vi "BRig_Host__Loop_Consumer_RunState__typeTrial__subtypeSelResult_parse__v2.vi"(0 "input_strCmd":string) -> (3 "output_selResult":bool, 4 "output_nTrial":u16, 6 "output_sSelection":u16, 8 "output_tSelection":u16, 10 "output_iReward_or_iError":u16, 13 "output_trig_l2":u16, 14 "output_trig_l1":u16, 15 "output_LorR":u16)   [LabVIEW 2014]
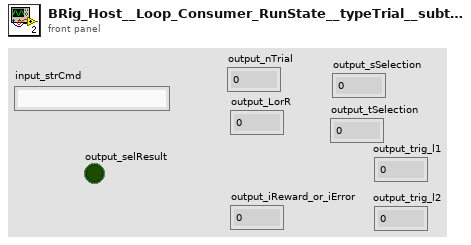
[diagram p1: front panel]
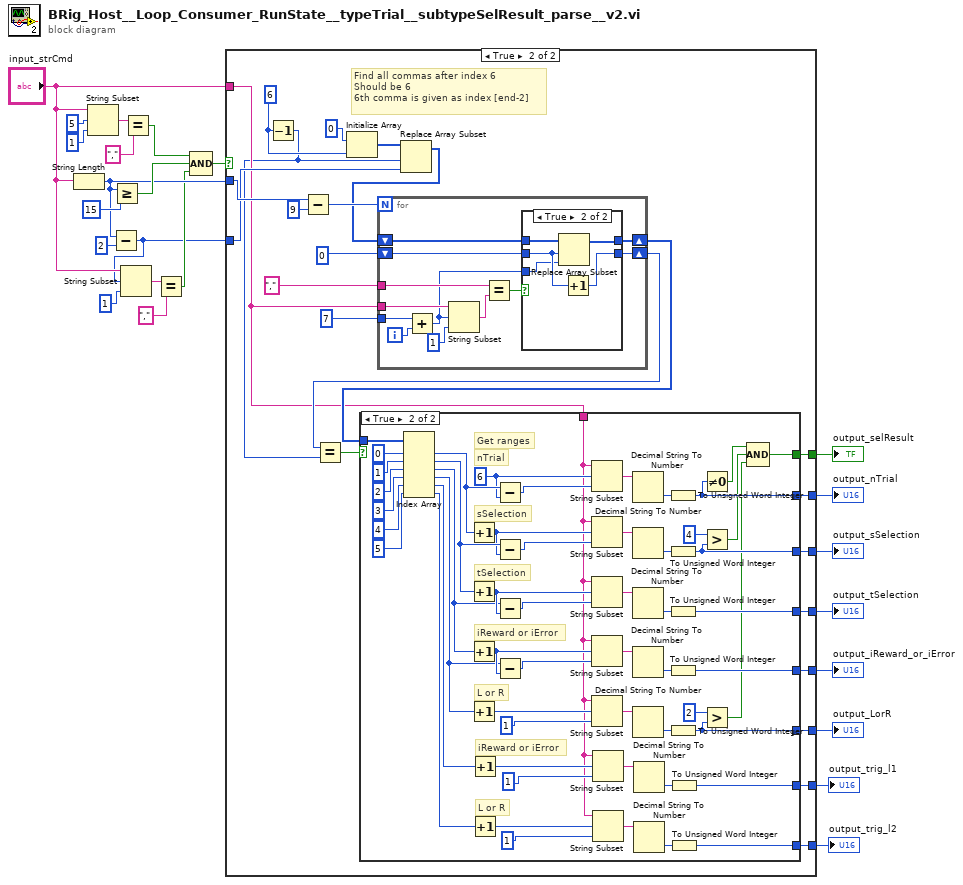
[diagram p0: block diagram]
diagram:
  n1 = String Length(string="input_strCmd") -> (length=w12:i32)
  n2 = String Subset(string="input_strCmd", offset (0)=5, length (rest)=1 ("offset (0)")) -> (substring=w22:string)
  n3 = Subtract(x=w12, y=2) -> (x-y=w9:i32)
  n4 = Greater Or Equal?(x=w12, y=15) -> (x >= y?=w19:bool)
  n5 = String Subset(string="input_strCmd", offset (0)=w9, length (rest)=1 ("offset (0)")) -> (substring=w14:string)
  n6 = Equal?(x=w22, y=",") -> (x = y?=w18:bool)
  n7 = Equal?(x=w14, y=",") -> (x = y?=w10:bool)
  n8 = Compound Arithmetic op=AND(w18, w19, w10) -> (w17:bool)
  n9 = case shown="True" w17 {
    tunnel: "input_strCmd" -> [_ w36]
    tunnel: w12 -> [_ w46]
    tunnel: w9 -> [_ w38]
    tunnel: [_ w34] -> w8
    tunnel: [_ w33] -> w7
    tunnel: [_ w32] -> w6
    tunnel: [_ w31] -> w5
    tunnel: [_ w30] -> w4
    tunnel: [_ w29] -> w3
    tunnel: [_ w26] -> w2
    tunnel: [_ w25] -> w1
    frame False {
    }
    frame True {
      w28 = 6 ("dimension size")
      # "Find all commas after index 6\nShould be 6\n6th comma is given as index [end-2]"
      n10 = Decrement(x=w28) -> (x-1=w27:i32)
      n11 = Subtract(x=w46, y=9) -> (x-y=w45:i32)
      n12 = Initialize Array(0 ("element"), w28) -> (w40:i32[])
      n13 = Replace Array Subset(array=w40, new element=w38, index=w27) -> (w39:i32[])
      n14 = for {
        N: w45 -> [_]
        tunnel: w36 -> [w114]
        tunnel: "," ("y") -> [w112]
        tunnel: 7 ("element") -> [w110]
        shift-right: [w104] -> w41
        shift-left: 0 ("element") -> [w106]
        shift-right: [w105] -> w37
        shift-left: w39 -> [w107]
        i -> [w111]
        n15 = Add(x=w110, y=w111) -> (x+y=w108:i32)
        n16 = String Subset(string=w114, offset (0)=w108, length (rest)=1 ("offset (0)")) -> (substring=w113:string)
        n17 = Equal?(x=w112, y=w113) -> (x = y?=w109:bool)
        n18 = case shown="True" w109 {
          tunnel: w108 -> [_ w119]
          tunnel: w107 -> [w117 w122]
          tunnel: w106 -> [w116 w120]
          tunnel: [w117 w121] -> w105
          tunnel: [w116 w118] -> w104
          frame False {
          }
          frame True {
            n19 = Replace Array Subset(array=w122, new element=w119, index=w120) -> (w121:i32[])
            n20 = Increment(x=w120) -> (x+1=w118:i32)
          }
        }
      }
      n21 = Equal?(x=w41, y=w27) -> (x = y?=w35:bool)
      n22 = case shown="True" w35 {
        tunnel: w37 -> [_ w103]
        tunnel: w36 -> [_ w51]
        tunnel: [_ w72] -> w34
        tunnel: [_ w68] -> w33
        tunnel: [_ w71] -> w32
        tunnel: [_ w82] -> w31
        tunnel: [_ w81] -> w30
        tunnel: [_ w64] -> w29
        tunnel: [_ w50] -> w26
        tunnel: [_ w49] -> w25
        frame False {
        }
        frame True {
          w79 = 6 ("y")
          # "L or R"
          # "iReward or iError"
          # "L or R"
          # "iReward or iError"
          # "tSelection"
          # "sSelection"
          # "nTrial"
          # "Get ranges"
          n23 = Index Array(array=w103, index #1=0 ("index"), index #2=1 ("index"), index #3=2 ("index"), index #4=3 ("index"), index #5=4 ("index"), index #6=5 ("index")) -> (element #1=w80:i32, element #2=w78:i32, element #3=w73:i32, element #4=w75:i32, element #5=w54:i32, element #6=w53:i32)
          n24 = Increment(x=w80) -> (x+1=w77:i32)
          n25 = Increment(x=w78) -> (x+1=w74:i32)
          n26 = Increment(x=w73) -> (x+1=w76:i32)
          n27 = Increment(x=w75) -> (x+1=w94:i32)
          n28 = Increment(x=w54) -> (x+1=w55:i32)
          n29 = Increment(x=w53) -> (x+1=w61:i32)
          n30 = Subtract(x=w80, y=w79) -> (x-y=w98:i32)
          n31 = Subtract(x=w78, y=w77) -> (x-y=w97:i32)
          n32 = Subtract(x=w73, y=w74) -> (x-y=w96:i32)
          n33 = Subtract(x=w75, y=w76) -> (x-y=w95:i32)
          n34 = String Subset(string=w51, offset (0)=w79, length (rest)=w98) -> (substring=w92:string)
          n35 = String Subset(string=w51, offset (0)=w77, length (rest)=w97) -> (substring=w91:string)
          n36 = String Subset(string=w51, offset (0)=w74, length (rest)=w96) -> (substring=w90:string)
          n37 = String Subset(string=w51, offset (0)=w76, length (rest)=w95) -> (substring=w89:string)
          n38 = String Subset(string=w51, offset (0)=w94, length (rest)=1 ("y")) -> (substring=w88:string)
          n39 = String Subset(string=w51, offset (0)=w55, length (rest)=1 ("y")) -> (substring=w59:string)
          n40 = String Subset(string=w51, offset (0)=w61, length (rest)=1 ("y")) -> (substring=w58:string)
          n41 = Decimal String To Number(string=w92) -> (number=w87:i32)  [unwired: 2 in, 1 out]
          n42 = Decimal String To Number(string=w91) -> (number=w86:i32)  [unwired: 2 in, 1 out]
          n43 = Decimal String To Number(string=w90) -> (number=w85:i32)  [unwired: 2 in, 1 out]
          n44 = Decimal String To Number(string=w89) -> (number=w84:i32)  [unwired: 2 in, 1 out]
          n45 = Decimal String To Number(string=w88) -> (number=w83:i32)  [unwired: 2 in, 1 out]
          n46 = Decimal String To Number(string=w59) -> (number=w57:i32)  [unwired: 2 in, 1 out]
          n47 = Decimal String To Number(string=w58) -> (number=w56:i32)  [unwired: 2 in, 1 out]
          n48 = To Unsigned Word Integer(number=w87) -> (unsigned 16bit integer=w72:u16)
          n49 = To Unsigned Word Integer(number=w86) -> (unsigned 16bit integer=w71:u16)
          n50 = To Unsigned Word Integer(number=w85) -> (unsigned 16bit integer=w82:u16)
          n51 = To Unsigned Word Integer(number=w84) -> (unsigned 16bit integer=w81:u16)
          n52 = To Unsigned Word Integer(number=w83) -> (unsigned 16bit integer=w68:u16)
          n53 = To Unsigned Word Integer(number=w57) -> (unsigned 16bit integer=w50:u16)
          n54 = To Unsigned Word Integer(number=w56) -> (unsigned 16bit integer=w49:u16)
          n55 = Not Equal To 0?(x=w72) -> (x != 0?=w65:bool)
          n56 = Greater?(x=u16 4, y=w71) -> (0:w66:bool)
          n57 = Greater?(x=u16 2, y=w68) -> (0:w67:bool)
          n58 = Compound Arithmetic op=AND(w65, w66, w67) -> (w64:bool)
        }
      }
    }
  }
  "output_nTrial" <- w8
  "output_LorR" <- w7
  "output_selResult" <- w3
  "output_sSelection" <- w6
  "output_tSelection" <- w5
  "output_iReward_or_iError" <- w4
  "output_trig_l1" <- w2
  "output_trig_l2" <- w1
